vi "RenameControls.vi"(8 "error in (no error)":errorcluster, 9 "Output String":string, 10 "Input String":string, 11 "LVClassLibrary Refnum":refnum<vi>) -> (0 "error out":errorcluster, 3 "Library Refnum out":refnum<vi>)   [LabVIEW 2014, in "ClassRenamer.lvclass"]
uses:
  ClassRenamer.lvclass
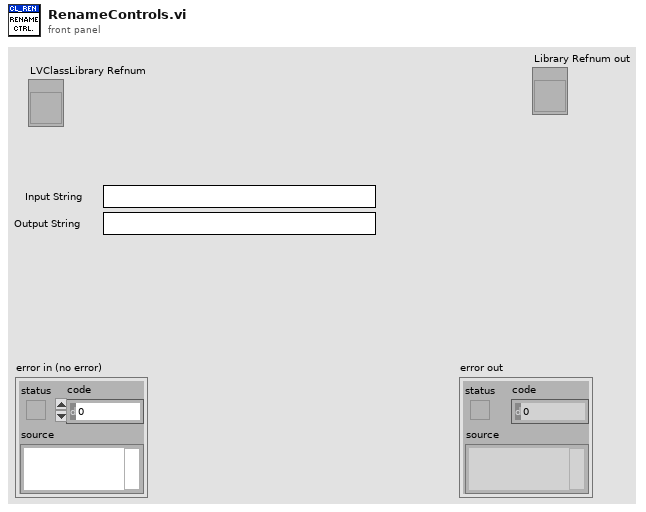
[diagram p1: front panel]
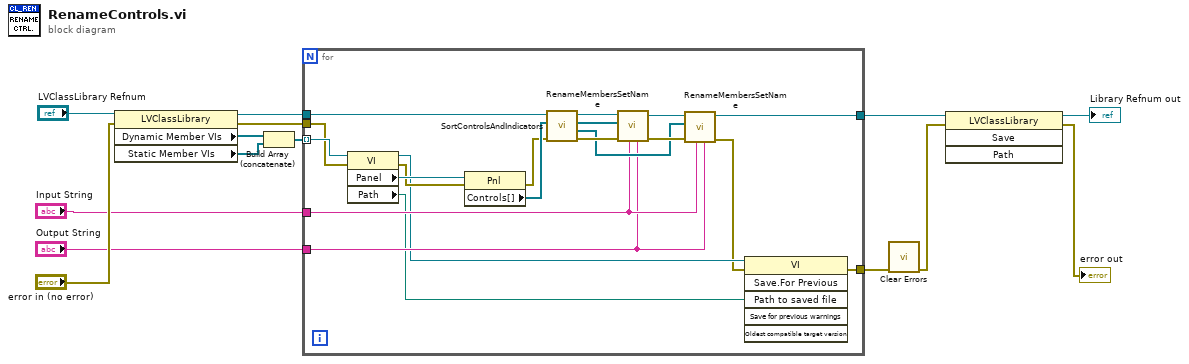
[diagram p0: block diagram]
diagram:
  n1 = property class="LVClassLibrary"(reference="LVClassLibrary Refnum", error in="error in (no error)") -> (reference out=w9:refnum<vi>, error out=w8:errorcluster, "Dynamic Member VIs"=w13:refnum<vi>[], "Static Member VIs"=w12:refnum<vi>[])
  n2 = Build Array (concatenate)(w13, w12) -> (w10:refnum<vi>[])
  n3 = for {
    tunnel: w10 -> [w33] mode=indexing
    tunnel: w9 -> [w30]
    tunnel: w8 -> [w32]
    tunnel: "Input String" -> [w21]
    tunnel: "Output String" -> [w20]
    tunnel: [w15] -> w5
    tunnel: [w19] -> w4
    n4 = property class="VI"(reference=w33, error in=w32) -> (reference out=w18:refnum<vi>, error out=w31:errorcluster, "Panel"=w34:refnum<vi>, "Path"=w17:path)
    n5 = property class="Pnl"(reference=w34, error in=w31) -> (error out=w28:errorcluster, "Controls[]"=w29:refnum<vi>[])  [unwired: 1 out]
    n6 = call "SortControlsAndIndicators.vi"("error in"=w28, "Controls[]"=w29, "LVClassLibrary Refnum"=w30) -> ("error out"=w25:errorcluster, "Controls"=w22:refnum<vi>[], "Indicators"=w26:refnum<vi>[], "Library Refnum out"=w27:refnum<vi>)  [unwired: 5 in]
    n7 = call "RenameMembersSetName.vi"("Output String"=w20, "Input String"=w21, "error in (no error)"=w25, "Controls"=w26, "LVClassLibrary Refnum"=w27) -> ("error out"=w23:errorcluster, "Library Refnum out"=w24:refnum<vi>)  [unwired: 5 in]
    n8 = call "RenameMembersSetName.vi"("Output String"=w20, "Input String"=w21, "error in (no error)"=w23, "Controls"=w22, "LVClassLibrary Refnum"=w24) -> ("error out"=w16:errorcluster, "Library Refnum out"=w19:refnum<vi>)  [unwired: 5 in]
    n9 = invoke class="VI" method="Save.For Previous"(reference=w18, error in=w16, "Path to saved file"=w17) -> (error out=w15:errorcluster)  [unwired: 3 in, 5 out]
  }
  n10 = call <vilib>:"Clear Errors.vi"("error in (no error)"=w5) -> ("error out"=w2:errorcluster)  [unwired: 5 in, 1 out]
  n11 = invoke class="LVClassLibrary" method="Save"(reference=w4, error in=w2) -> (reference out=→"Library Refnum out":refnum<vi>, error out=→"error out":errorcluster)  [unwired: 2 in, 2 out]
